vi "OffsetDialog.vi"(8 "error in (no error)":errorcluster) -> (0 "error out":errorcluster, 3 "Offest":dbl)   [LabVIEW 2015]
panel:
  in  "Discard":bool
  in  "OK":bool
  in  "Dialog":dbl=5.0 format="%#_g min"
  # "Enter time offset:"
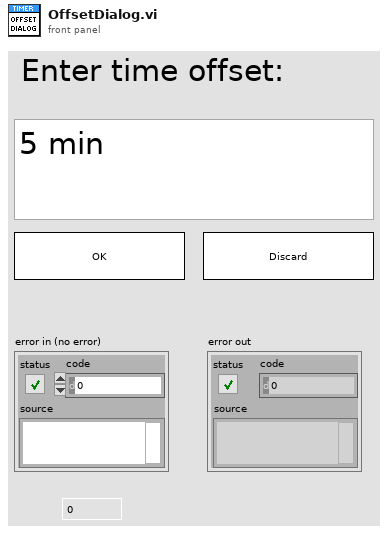
[diagram p1: front panel]
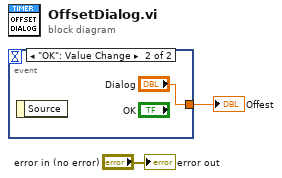
[diagram p0: block diagram]
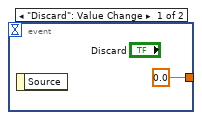
[diagram p2: hidden frame]
diagram:
  n1 = event shown="[1] \"OK\": Value Change" {
    selector: _ -> [_ _]
    dyn-events: _ -> [_ _]
    timeout: _ -> [_ _]
    tunnel: [0.0 "Dialog"] -> w2
    event "Discard": Value Change {
      n2 = event-data() -> ()  [unwired: 1 in, 1 out]
    }
    event "OK": Value Change {
      n3 = event-data() -> ()  [unwired: 1 in, 1 out]
    }
  }
  "Offest" <- w2
  "error out" <- "error in (no error)"
